vi "read_temperature.vi"(3 "VISA resource name":refnum<visa-resource-name> caption="VISA资源名称") -> (0 "温度":dbl, 1 "湿度":dbl)   [LabVIEW 2018]
uses:
  <vilib>/Instr/_visa.llb/VISA Configure Serial Port (Instr).vi
panel:
  out "Serial Settings:Number of Bytes at Serial Port":u32
  out "输出数组":u8[](array[numeric]) format="%x"
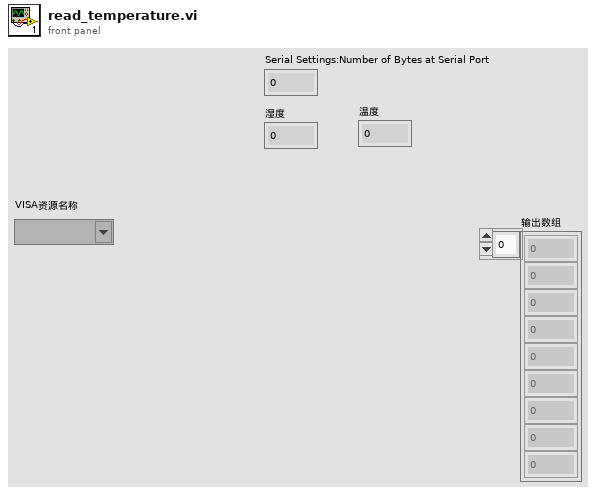
[diagram p1: front panel]
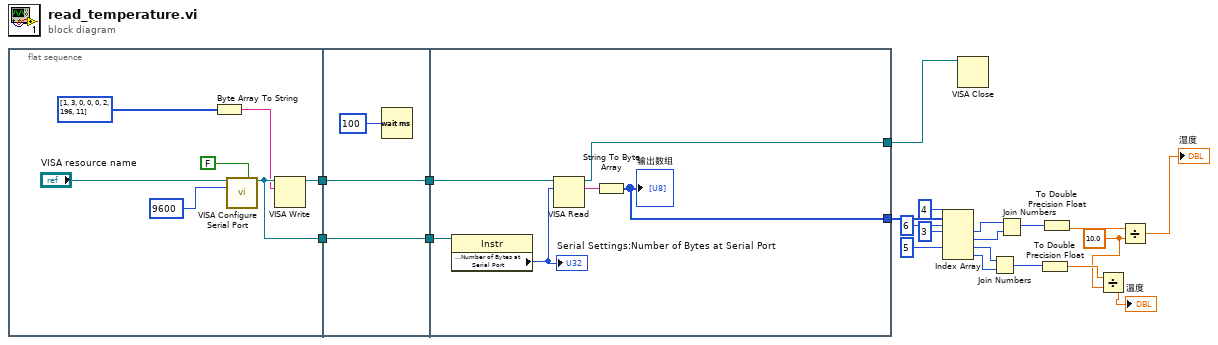
[diagram p0: block diagram]
diagram:
  w2 = 10.0 ("y")
  n1 = flat-sequence {
    tunnel: [w25] -> w21
    tunnel: [w24] -> w20
    tunnel: w21 -> [w31]
    tunnel: w20 -> [w30]
    tunnel: [w31] -> w19
    tunnel: [w30] -> w18
    tunnel: w19 -> [w34]
    tunnel: w18 -> [w35]
    tunnel: [w33] -> w17
    tunnel: [w32] -> w16
    frame #0 {
      n2 = Byte Array To String(unsigned byte array=u8[] [1, 3, 0, 0, 0, 2, 196, 11] ("输入数组 2")) -> (string=w23:string)
      n3 = call-poly "VISA Configure Serial Port"("VISA resource name"="VISA resource name", "Enable Termination\nChar (T)"=FALSE ("Enable Termination\nChar (T)"), "baud rate (9600)"=u32 9600) -> ("VISA resource name out"=w24:refnum<visa-resource-name>)  [unwired: 11 in, 1 out]
      n4 = VISA Write(VISA resource name=w24, write buffer=w23) -> (VISA resource name out=w25:refnum<visa-resource-name>)  [unwired: 1 in, 2 out]
    }
    frame #1 {
      n5 = Wait (ms)(milliseconds to wait=u32 100 ("等待时间（毫秒）")) -> ()  [unwired: 1 out]
    }
    frame #2 {
      n6 = property class="Instr"(reference=w35) -> ("Serial Settings:Number of Bytes at Serial Port"=w36:u32)  [unwired: 1 in, 2 out]
      "Serial Settings:Number of Bytes at Serial Port" <- w36
      n7 = VISA Read(VISA resource name=w34, byte count=w36) -> (VISA resource name out=w33:refnum<visa-resource-name>, read buffer=w37:string)  [unwired: 1 in, 2 out]
      n8 = String To Byte Array(string=w37) -> (unsigned byte array=w32:u8[])
      "输出数组" <- w32
    }
  }
  n9 = Index Array(array=w16, index #1=3 ("索引"), index #2=4 ("索引"), index #3=5 ("索引"), index #4=6 ("索引")) -> (element #1=w11:u8, element #2=w10:u8, element #3=w9:u8, element #4=w8:u8)
  n10 = VISA Close(VISA resource name=w17) -> ()  [unwired: 1 in, 1 out]
  n11 = Join Numbers(hi=w9, lo=w8) -> ((hi.lo)=w6:u16)
  n12 = Join Numbers(hi=w11, lo=w10) -> ((hi.lo)=w7:u16)
  n13 = To Double Precision Float(number=w6) -> (double precision float=w3:dbl)
  n14 = To Double Precision Float(number=w7) -> (double precision float=w5:dbl)
  n15 = Divide(x=w3, y=w2) -> (x/y=→"温度":dbl)
  n16 = Divide(x=w5, y=w2) -> (x/y=→"湿度":dbl)
